vi "SetList_ToString.vi"(1 "Column Names":string[](array[string]), 2 "Current  Variables":cluster{"Name":string, "Value":dbl}[](array[cluster]), 3 "Device Data":string[][](table)) -> (0 "Igor Inform String":string)   [LabVIEW 2013]
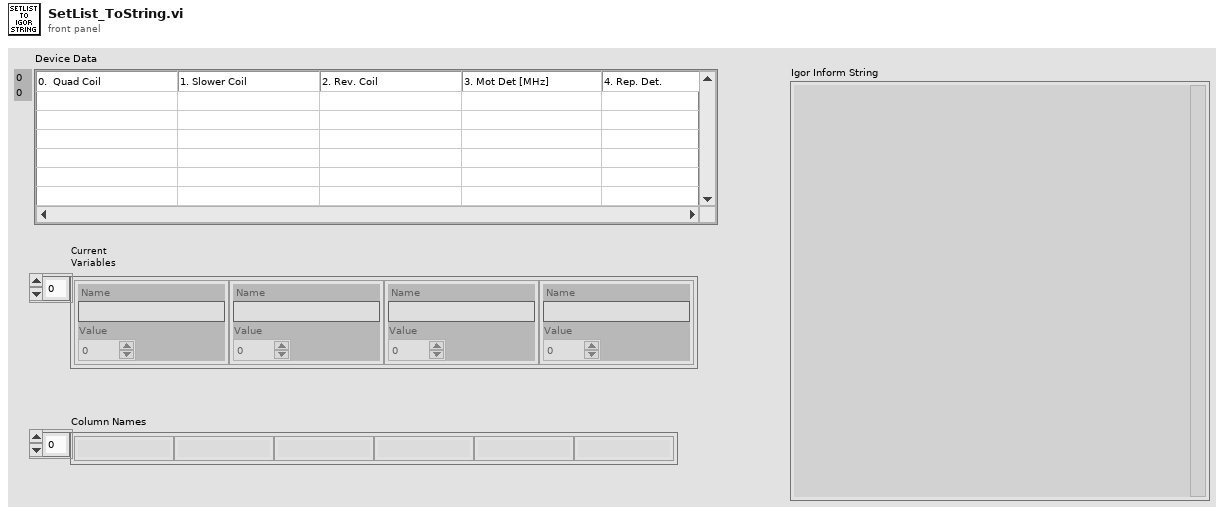
[diagram p1: front panel]
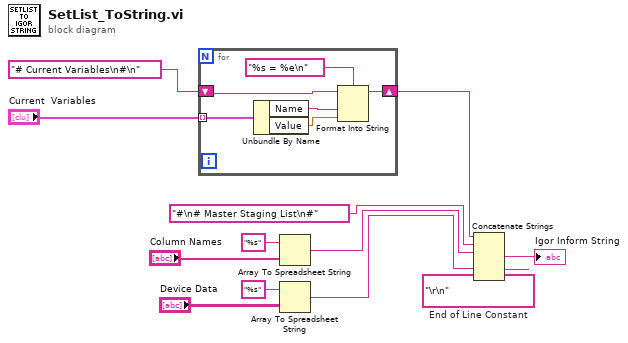
[diagram p0: block diagram]
diagram:
  w12 = "\r\n"  # End of Line Constant
  n1 = for {
    tunnel: "Current  Variables" -> [w15] mode=indexing
    shift-right: [w16] -> w2
    shift-left: "# Current Variables\n#\n" -> [w17]
    n2 = Unbundle By Name(w15) -> ("Name"=w14:string, "Value"=w13:dbl)
    n3 = Format Into String(format string="%s = %e\n", initial string=w17, w14, w13) -> (resulting string=w16:string)  [unwired: 1 in, 1 out]
  }
  n4 = Array To Spreadsheet String(array="Column Names", 3:"%s" ("delimiter (Tab)")) -> (spreadsheet string=w8:string)  [unwired: 1 in]
  n5 = Array To Spreadsheet String(array="Device Data", 3:"%s" ("delimiter (Tab)")) -> (spreadsheet string=w11:string)  [unwired: 1 in]
  n6 = Concatenate Strings(w2, "#\n# Master Staging List\n#", w8, w12, w11, w12) -> (→"Igor Inform String":string)
